vi "1_elements_of_labview.vi"() -> ()   [LabVIEW 2015]
uses:
  <vilib>/measure/NI_MABase.lvlib
panel:
  out "signal out":waveform(dbl) caption="신호 출력"
  out "양의 피크":dbl
  out "음의 피크":dbl
  out "y":dbl
  in  "x":dbl
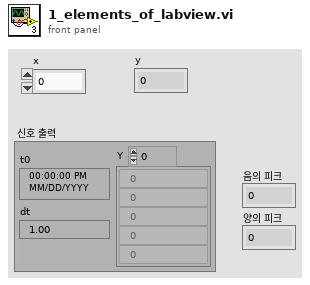
[diagram p1: front panel]
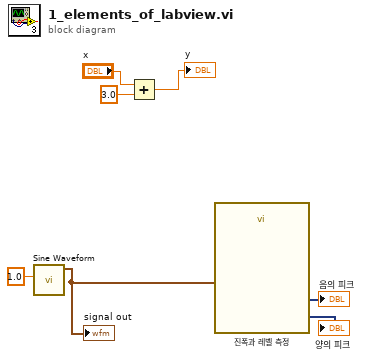
[diagram p0: block diagram]
diagram:
  n1 = call <vilib>:"Sine Waveform.vi"("amplitude"=1.0) -> ("signal out"=w2:waveform(dbl))  [unwired: 9 in, 1 out]
  "signal out" <- w2
  n2 = Add(x="x", y=3.0) -> (x+y=→"y":dbl)
  n3 = call "진폭과 레벨 측정"("Signals"=w2) -> ("Negative Peak"=→"음의 피크":dynamicdata, "Positive Peak"=→"양의 피크":dynamicdata)  [unwired: 12 in, 1 out]
